vi "Tank Controll sim.vi"() -> ()   [LabVIEW 2017]
uses:
  <vilib>/addons/control/pid/pid.llb/PID (DBL).vi
  <vilib>/Waveform/DWDTOps.llb/DWDT Analog to Digital.vi
  <vilib>/Waveform/DWDTOps.llb/DWDT Digital to Boolean Array.vi
  <vilib>/measure/NI_MABase.lvlib
  <vilib>/addons/control/pid/NI_PID_pid.lvlib
panel:
  out "Ready to Start":bool
  out "Temp":string
  in  "Heater\nControll":bool
  out "PWM - Duty Cycle (%)":dbl format="%.2f"
  in  "PID gains":T1={"proportional gain (Kc)"=1.0, "integral time (Ti, min)"=0.01, "derivative time (Td, min)"=0.0} {"derivative time (Td, min)" format="%.3f"; "integral time (Ti, min)" format="%.3f"; "proportional gain (Kc)" format="%.3f"}
  out "Heater on":bool
  out "Setpoint two high":string
  out "Setpoint two high":string
  out "String 3":string
  in  "Feed Tank":dbl(slide) scale=0.0..20.0
  in  "Temp. Setpoint":dbl
  in  "Tank 2 \nTemp.":dbl(slide) scale=15.0..100.0
  out "Tank 2 Level":string
  out "Tank 1 Level":string
  in  "Cycle Stop":bool
  in  "Start":bool
  in  "Position 2":bool
  in  "Position 1":bool
  out "Conveyor":bool
  out "Drop 2":bool
  out "Drop 1":bool
  out "Fill Two":bool
  out "Fill One":bool
  in  "Fill\nControll":bool
  in  "Setpoint  2":dbl
  in  "Tank 2":dbl(slide) scale=0.0..20.0
  out "Pump on":bool
  in  "Setpoint":dbl
  in  "stop":bool
  in  "Tank 1":dbl(slide) scale=0.0..20.0
  # "Auto"
  # "Manual"
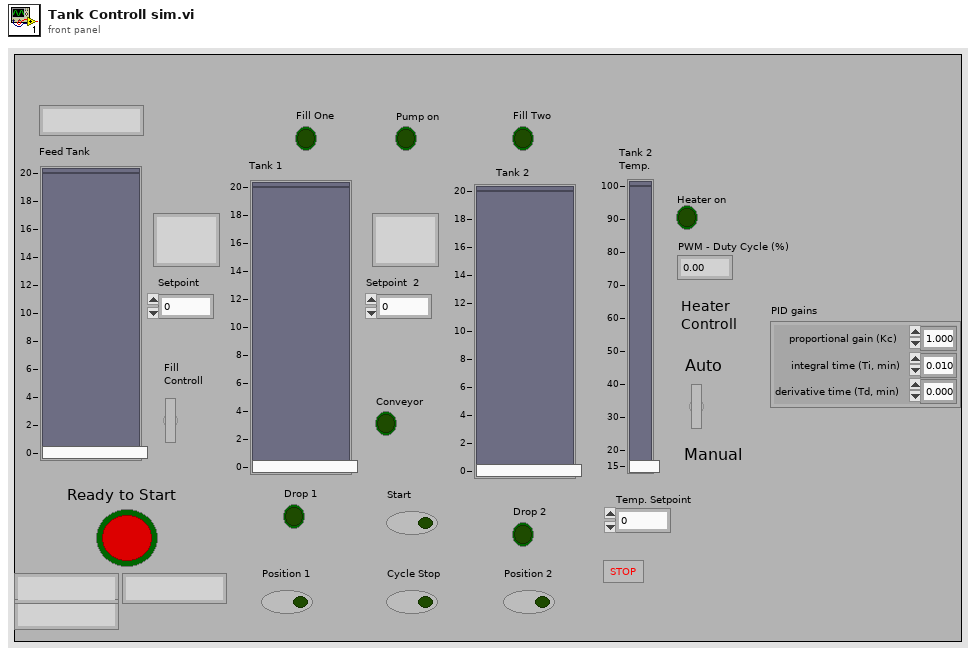
[diagram p1: front panel]
types:
  T1 = cluster{"proportional gain (Kc)":dbl, "integral time (Ti, min)":dbl, "derivative time (Td, min)":dbl}
  T2 = enum16{"Wait For Start", "Move Tank 1", "Fill One", "Move Tank 2", "Fill Two", "Move to Stop", "Stop All"}
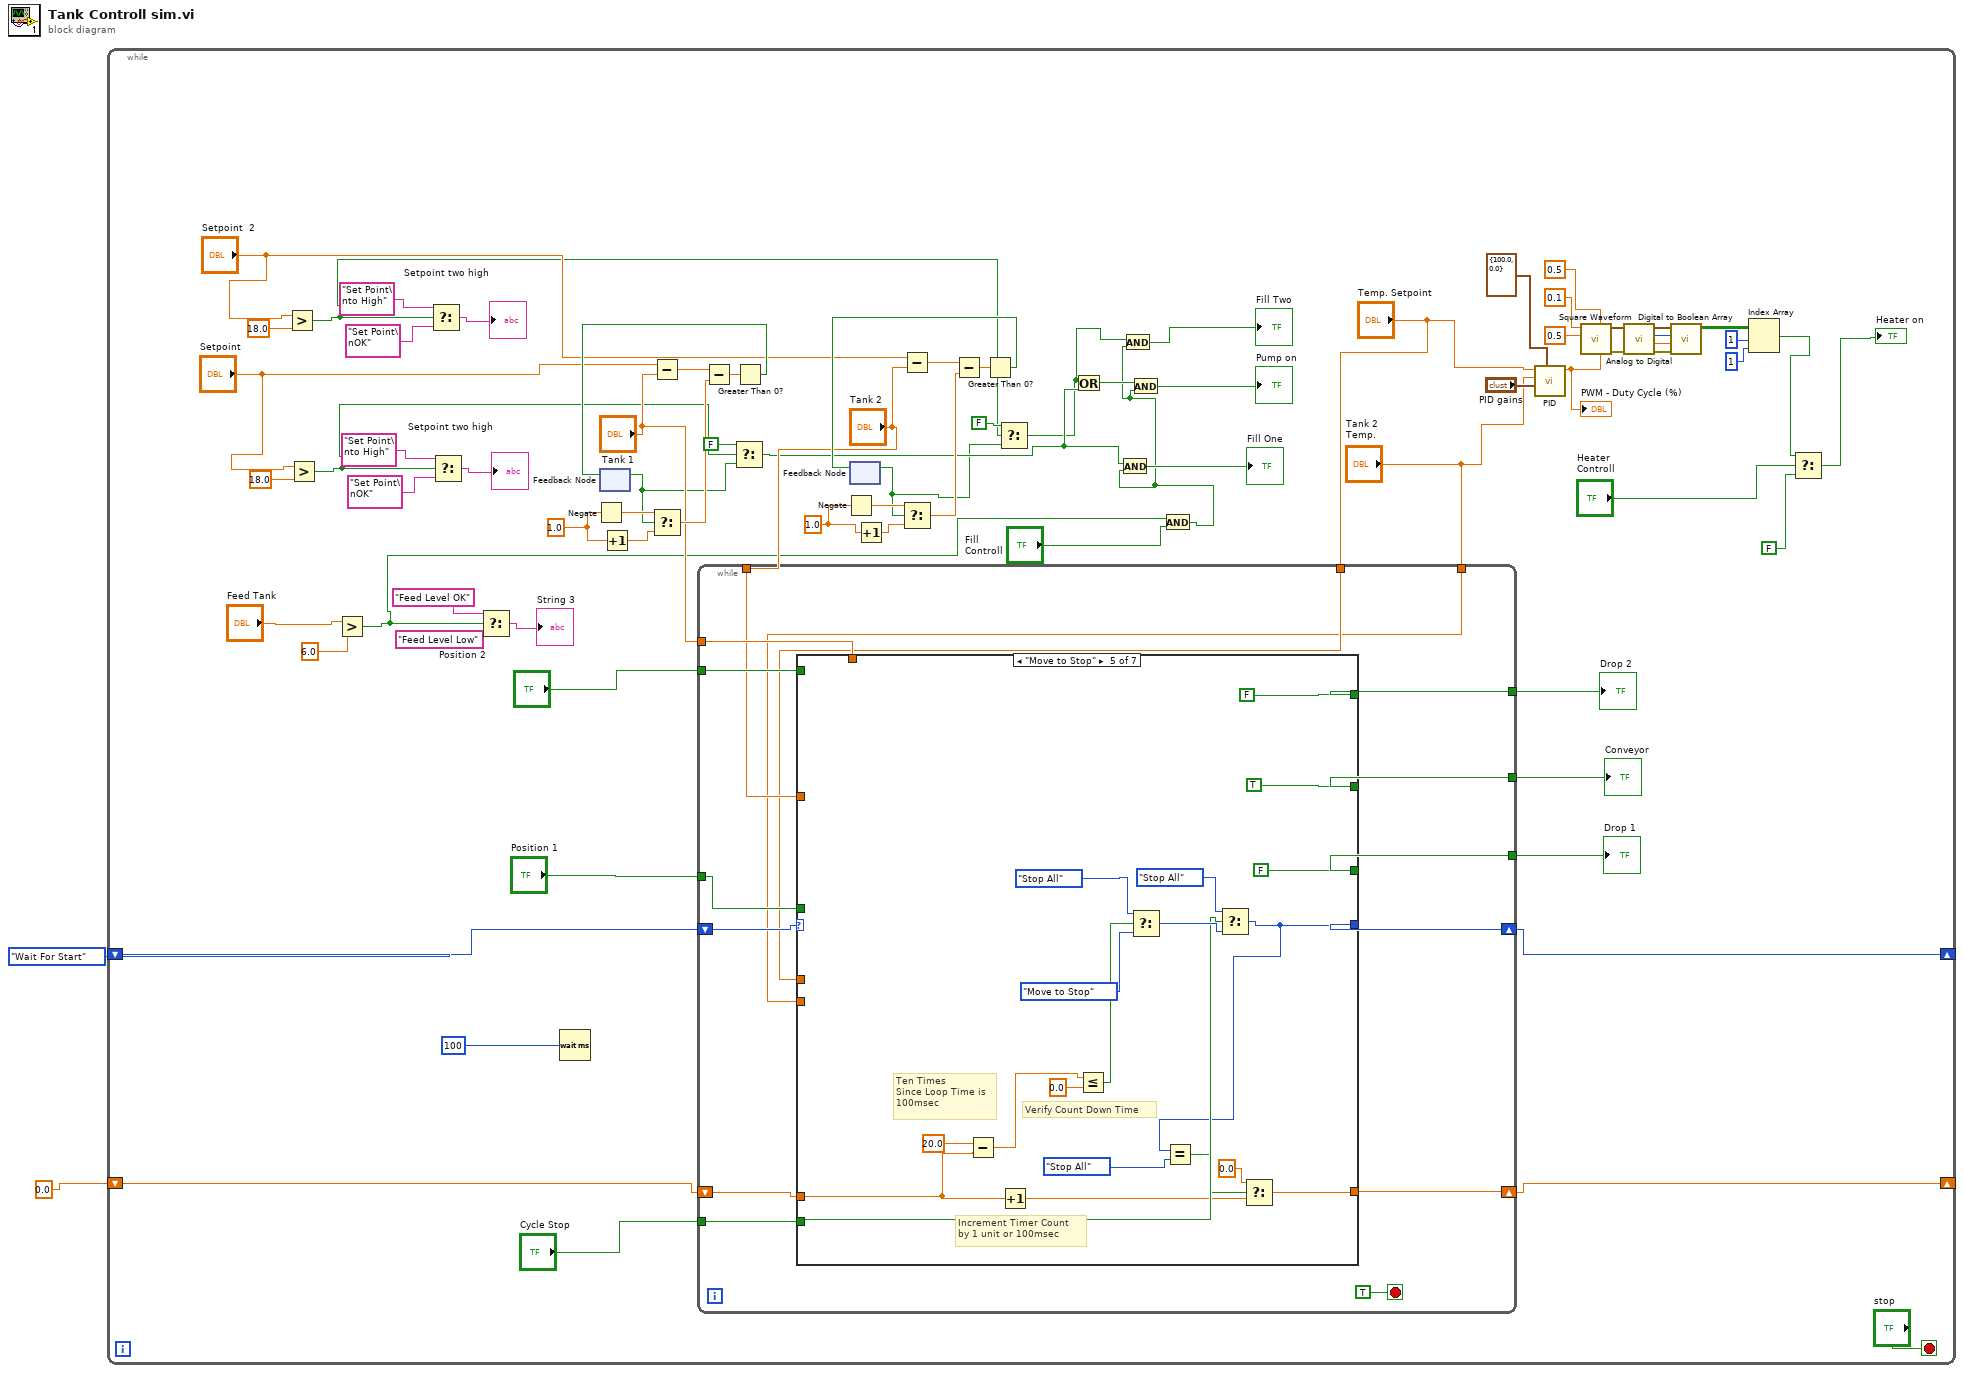
[diagram p0: block diagram]
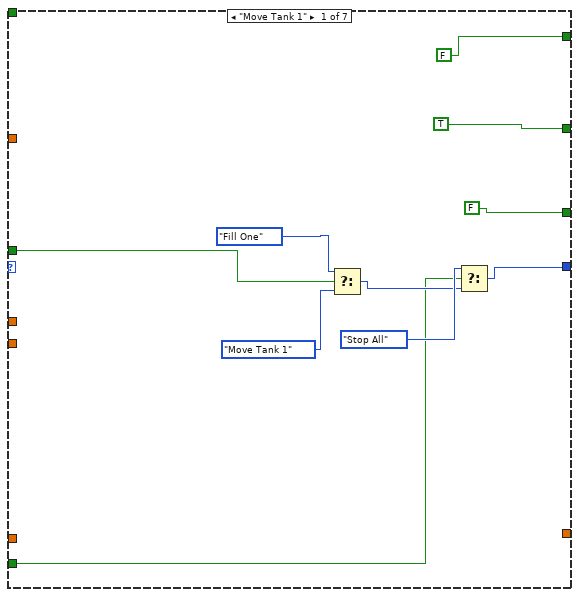
[diagram p2: hidden frame]
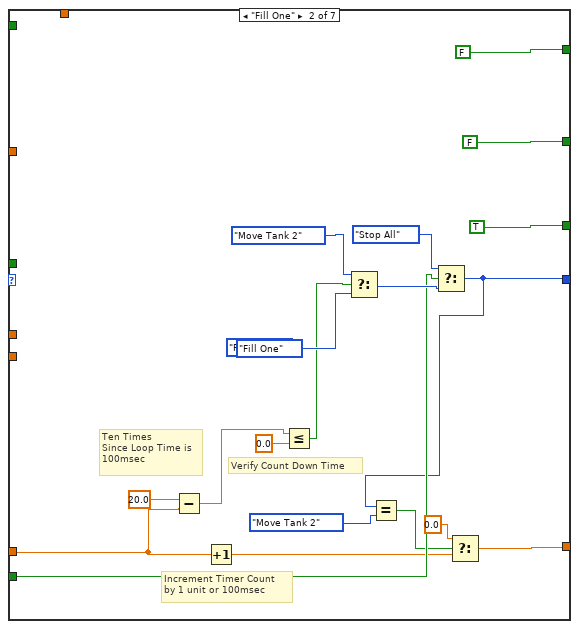
[diagram p3: hidden frame]
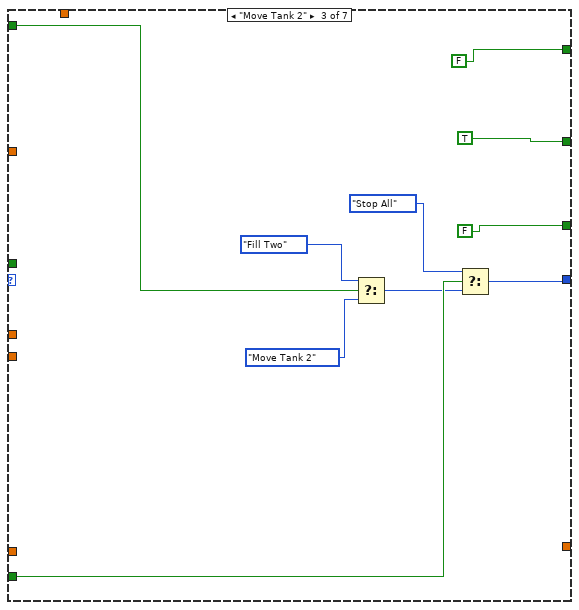
[diagram p4: hidden frame]
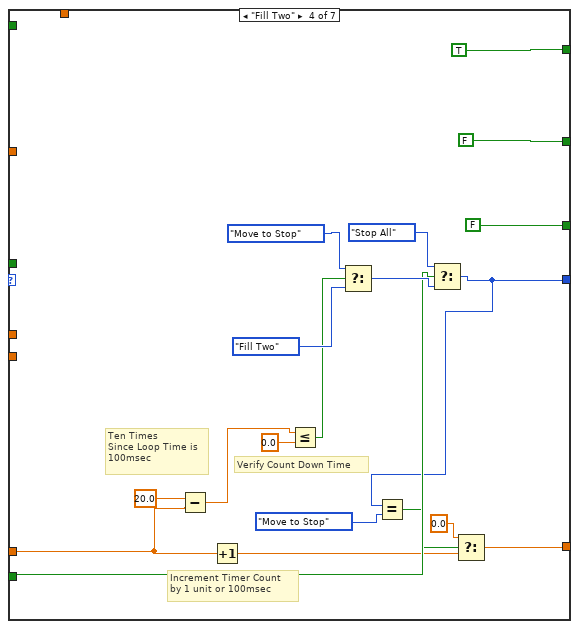
[diagram p5: hidden frame]
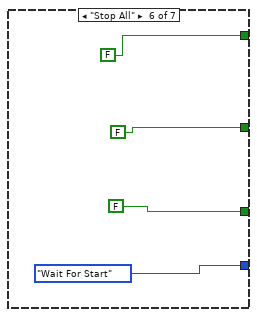
[diagram p6: hidden frame]
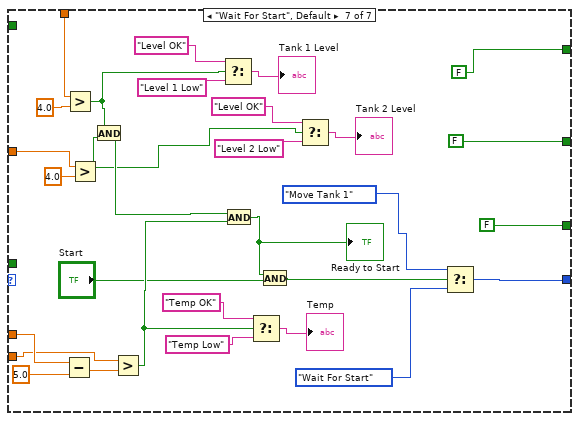
[diagram p7: hidden frame]
diagram:
  n1 = while {
    shift-right: [w60] -> _
    shift-left: T2."Wait For Start" -> [w61]
    shift-right: [w57] -> _
    shift-left: 0.0 ("Time Target (s)") -> [w58]
    stop <- "stop" stop-if-true
    w53 = 1.0 ("y")
    w56 = 1.0 ("y")
    n2 = Greater?(x="Setpoint  2", y=18.0) -> (0:w27:bool)
    n3 = Greater?(x="Setpoint", y=18.0) -> (0:w36:bool)
    n4 = Greater?(x="Feed Tank", y=6.0) -> (0:w42:bool)
    n5 = Select(t="Set Point\nto High", s=w27, f="Set Point\nOK") -> (s? t:f=→"Setpoint two high":string)
    n6 = Select(t="Set Point\nto High", s=w36, f="Set Point\nOK") -> (s? t:f=→"Setpoint two high":string)
    n7 = Select(t="Feed Level OK", s=w42, f="Feed Level Low") -> (s? t:f=→"String 3":string)
    n8 = Wait (ms)(milliseconds to wait=u32 100) -> ()  [unwired: 1 out]
    n9 = Negate(x=w56) -> (-x=w75:dbl)
    n10 = feedback #1() -> (w35:bool)  [unwired: 1 in]
    n11 = Increment(x=w56) -> (x+1=w55:dbl)
    n12 = Subtract(x="Setpoint", y="Tank 1") -> (x-y=w78:dbl)
    n13 = Select(t=w75, s=w35, f=w55) -> (s? t:f=w79:dbl)
    n14 = while {
      tunnel: "Position 2" -> [w89]
      tunnel: "Position 1" -> [w93]
      shift-right: [w95] -> w60
      shift-left: w61 -> [w94]
      tunnel: [w92] -> w64
      tunnel: [w91] -> w63
      tunnel: [w90] -> w62
      tunnel: "Cycle Stop" -> [w88]
      shift-right: [w86] -> w57
      shift-left: w58 -> [w87]
      tunnel: "Tank 1" -> [w85]
      tunnel: "Tank 2" -> [w84]
      tunnel: "Temp. Setpoint" -> [w83]
      tunnel: "Tank 2 \nTemp." -> [w82]
      stop <- TRUE stop-if-true
      n15 = case shown="\"Move to Stop\"" w94 {
        tunnel: [w98 w107 w126 w137 w156 T2."Wait For Start" w205] -> w95
        tunnel: [FALSE ("Drop 2") FALSE ("Drop 2") FALSE ("Drop 2") TRUE ("Drop 2") FALSE ("Drop 2") FALSE ("Drop 2") FALSE ("Drop 2")] -> w92
        tunnel: [TRUE ("Drop 2") FALSE ("Drop 2") TRUE ("Drop 2") FALSE ("Drop 2") TRUE ("Drop 2") FALSE ("Drop 2") FALSE ("Drop 2")] -> w91
        tunnel: [FALSE ("Drop 2") TRUE ("Drop 2") FALSE ("Drop 2") FALSE ("Drop 2") FALSE ("Drop 2") FALSE ("Drop 2") FALSE ("Drop 2")] -> w90
        tunnel: w93 -> [w101 _ _ _ _ _ _]
        tunnel: w89 -> [_ _ w130 _ _ _ _]
        tunnel: w88 -> [w97 w118 w129 w150 w169 _ _]
        tunnel: w87 -> [_ w109 _ w140 w159 _ _]
        tunnel: [_ w110 _ w136 w155 _ _] -> w86
        tunnel: w85 -> [_ _ _ _ _ _ w198]
        tunnel: w84 -> [_ _ _ _ _ _ w197]
        tunnel: w83 -> [_ _ _ _ _ _ w182]
        tunnel: w82 -> [_ _ _ _ _ _ w181]
        frame "Move Tank 1" {
          n16 = Select(t=T2."Fill One", s=w101, f=T2."Move Tank 1") -> (s? t:f=w99:T2)
          n17 = Select(t=T2."Stop All", s=w97, f=w99) -> (s? t:f=w98:T2)
        }
        frame "Fill One" {
          (unwired) T2."Fill One"
          # "Increment Timer Count \nby 1 unit or 100msec"
          # "Verify Count Down Time"
          # "Ten Times\nSince Loop Time is\n100msec"
          n18 = Subtract(x=20.0, y=w109) -> (x-y=w117:dbl)
          n19 = Increment(x=w109) -> (x+1=w113:dbl)
          n20 = Less Or Equal?(x=w117, y=0.0) -> (x <= y?=w108:bool)
          n21 = Select(t=T2."Move Tank 2", s=w108, f=T2."Fill One") -> (s? t:f=w120:T2)
          n22 = Select(t=T2."Stop All", s=w118, f=w120) -> (s? t:f=w107:T2)
          n23 = Equal?(x=w107, y=T2."Move Tank 2") -> (x = y?=w114:bool)
          n24 = Select(t=0.0 ("y"), s=w114, f=w113) -> (s? t:f=w110:dbl)
        }
        frame "Move Tank 2" {
          n25 = Select(t=T2."Fill Two", s=w130, f=T2."Move Tank 2") -> (s? t:f=w127:T2)
          n26 = Select(t=T2."Stop All", s=w129, f=w127) -> (s? t:f=w126:T2)
        }
        frame "Fill Two" {
          # "Increment Timer Count \nby 1 unit or 100msec"
          # "Verify Count Down Time"
          # "Ten Times\nSince Loop Time is\n100msec"
          n27 = Subtract(x=20.0, y=w140) -> (x-y=w146:dbl)
          n28 = Increment(x=w140) -> (x+1=w142:dbl)
          n29 = Less Or Equal?(x=w146, y=0.0) -> (x <= y?=w138:bool)
          n30 = Select(t=T2."Move to Stop", s=w138, f=T2."Fill Two") -> (s? t:f=w153:T2)
          n31 = Select(t=T2."Stop All", s=w150, f=w153) -> (s? t:f=w137:T2)
          n32 = Equal?(x=w137, y=T2."Move to Stop") -> (x = y?=w143:bool)
          n33 = Select(t=0.0 ("y"), s=w143, f=w142) -> (s? t:f=w136:dbl)
        }
        frame "Move to Stop" {
          # "Increment Timer Count \nby 1 unit or 100msec"
          # "Verify Count Down Time"
          # "Ten Times\nSince Loop Time is\n100msec"
          n34 = Subtract(x=20.0, y=w159) -> (x-y=w165:dbl)
          n35 = Increment(x=w159) -> (x+1=w161:dbl)
          n36 = Less Or Equal?(x=w165, y=0.0) -> (x <= y?=w157:bool)
          n37 = Select(t=T2."Stop All", s=w157, f=T2."Move to Stop") -> (s? t:f=w172:T2)
          n38 = Select(t=T2."Stop All", s=w169, f=w172) -> (s? t:f=w156:T2)
          n39 = Equal?(x=w156, y=T2."Stop All") -> (x = y?=w162:bool)
          n40 = Select(t=0.0 ("y"), s=w162, f=w161) -> (s? t:f=w155:dbl)
        }
        frame "Stop All" {
        }
        frame "Wait For Start", Default {
          n41 = Subtract(x=w182, y=5.0) -> (x-y=w183:dbl)
          n42 = Greater?(x=w198, y=4.0) -> (0:w194:bool)
          n43 = Greater?(x=w197, y=4.0) -> (0:w189:bool)
          n44 = And(x=w194, y=w189) -> (x .and. y?=w199:bool)
          n45 = Greater?(x=w181, y=w183) -> (0:w180:bool)
          n46 = Select(t="Level OK", s=w194, f="Level 1 Low") -> (s? t:f=→"Tank 1 Level":string)
          n47 = And(x=w199, y=w180) -> (x .and. y?=w178:bool)
          "Ready to Start" <- w178
          n48 = Select(t="Temp OK", s=w180, f="Temp Low") -> (s? t:f=→"Temp":string)
          n49 = And(x=w178, y="Start") -> (x .and. y?=w185:bool)
          n50 = Select(t="Level OK", s=w189, f="Level 2 Low") -> (s? t:f=→"Tank 2 Level":string)
          n51 = Select(t=T2."Move Tank 1", s=w185, f=T2."Wait For Start") -> (s? t:f=w205:T2)
        }
      }
    }
    "Drop 2" <- w64
    "Conveyor" <- w63
    "Drop 1" <- w62
    n52 = Subtract(x=w78, y=w79) -> (x-y=w80:dbl)
    n53 = Select(t=FALSE, s=w36, f=w35) -> (s? t:f=w26:bool)
    n54 = Greater Than 0?(x=w80) -> (x > 0?=w77:bool)
    n55 = feedback-in #1(w77) -> ()
    n56 = Negate(x=w53) -> (-x=w54:dbl)
    n57 = feedback #2() -> (w25:bool)  [unwired: 1 in]
    n58 = Increment(x=w53) -> (x+1=w52:dbl)
    n59 = Subtract(x="Setpoint  2", y="Tank 2") -> (x-y=w72:dbl)
    n60 = Select(t=w54, s=w25, f=w52) -> (s? t:f=w73:dbl)
    n61 = Subtract(x=w72, y=w73) -> (x-y=w74:dbl)
    n62 = Greater Than 0?(x=w74) -> (x > 0?=w71:bool)
    n63 = feedback-in #2(w71) -> ()
    n64 = Select(t=FALSE, s=w27, f=w25) -> (s? t:f=w24:bool)
    n65 = Or(x=w24, y=w26) -> (x .or. y?=w70:bool)
    n66 = And(x=w42, y="Fill\nControll") -> (x .and. y?=w44:bool)
    n67 = And(x=w26, y=w44) -> (x .and. y?=→"Fill One":bool)
    n68 = And(x=w24, y=w44) -> (x .and. y?=→"Fill Two":bool)
    n69 = And(x=w70, y=w44) -> (x .and. y?=→"Pump on":bool)
    n70 = call-poly <vilib>:"PID.vi"("output range"=cluster{"output high":dbl, "output low":dbl} {"output high"=100.0, "output low"=0.0}, "PID gains"="PID gains", "process variable"="Tank 2 \nTemp.", "setpoint"="Temp. Setpoint") -> ("output"=w11:dbl)  [unwired: 6 in, 1 out]
    "PWM - Duty Cycle (%)" <- w11
    n71 = call <vilib>:"Square Waveform.vi"("duty cycle (%)"=w11, "offset"=0.5, "amplitude"=0.5, "frequency"=0.1) -> ("error out"=w17:errorcluster, "signal out"=w9:waveform(dbl))  [unwired: 6 in]
    n72 = call-poly <vilib>:"Analog to Digital.vi"("error in (no error)"=w17, "analog waveform"=w9) -> ("error out"=w18:errorcluster, "full-scale range (out)"=w19:dbl, "resolution (out)"=w20:i32, "digital waveform"=w10:digitalwaveform)  [unwired: 6 in]
    n73 = call-poly <vilib>:"Digital to Boolean Array.vi"("error in (no error)"=w18, "mode"=w19, "response on error"=w20, "digital waveform"=w10) -> ("boolean array"=w23:bool[][])  [unwired: 6 in, 1 out]
    n74 = Index Array(array=w23, index (row)=1, index (col)=1 ("disabled index (col)")) -> (element=w7:bool)
    n75 = Select(t=w7, s="Heater\nControll", f=FALSE) -> (s? t:f=→"Heater on":bool)
  }
